vi "Start Download.vi"(5 "Overall Status":refnum<vi>, 7 "Itemized Status":refnum<vi>, 8 "Error In":errorcluster, 11 "Dependecy Config":T2) -> (0 "Error Out":errorcluster, 2 "Install State":T1(ring), 3 "Dependecy Config":T2)   [LabVIEW 2011, in "LVH-Toolbox.lvlib" / "Installer Tools.lvlib"]
uses:
  Installer Tools.lvlib
  Type Defs/Dependency Config.ctl
  Type Defs/Dependecy.ctl
  Common/Private/Web/Type Defs/Download Task.ctl
  Common/LVH-Common.lvlib
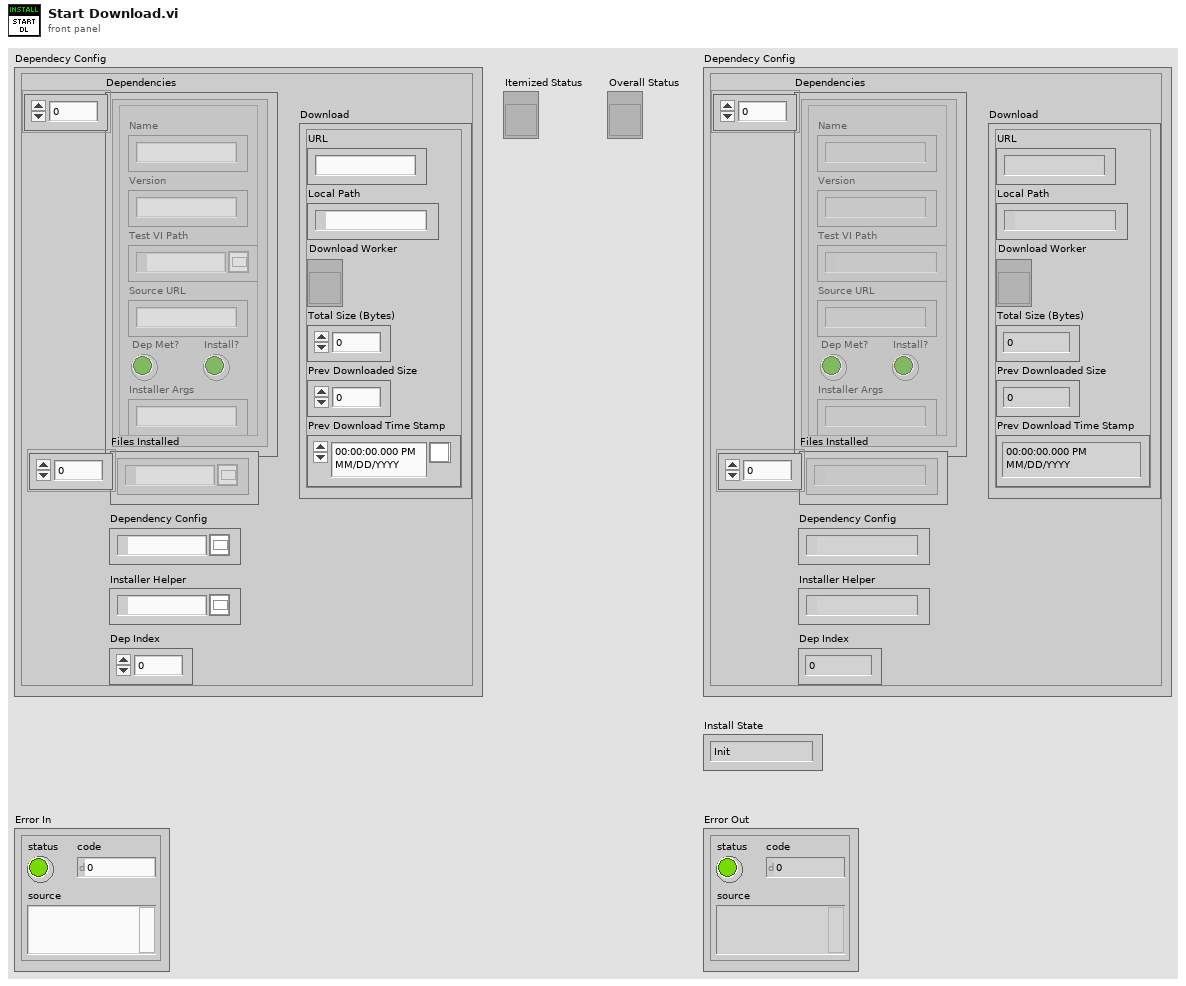
[diagram p1: front panel]
types:
  T1 = enum16{"Init", "Start DL", "Downloading", "DL Complete", "Done"}
  T2 = typedef "LVH-Toolbox.lvlib/Installer Tools.lvlib/Dependency Config.ctl" = cluster{"Dependencies":T3[], "Files Installed":path[], "Dependency Config":path, "Installer Helper":path, "Dep Index":i32, "Download":T4}
  T3 = typedef "LVH-Toolbox.lvlib/Installer Tools.lvlib/Dependecy.ctl" = cluster{"Name":string, "Version":string, "Test VI Path":path, "Source URL":string, "Dep Met?":bool, "Install?":bool, "Installer Args":string}
  T4 = typedef "LVH-Toolbox.lvlib/LVH-Common.lvlib/Download Task.ctl" = cluster{"URL":string, "Local Path":path, "Download Worker":refnum<vi>, "Total Size (Bytes)":u64, "Prev Downloaded Size":u64, "Prev Download Time Stamp":timestamp}
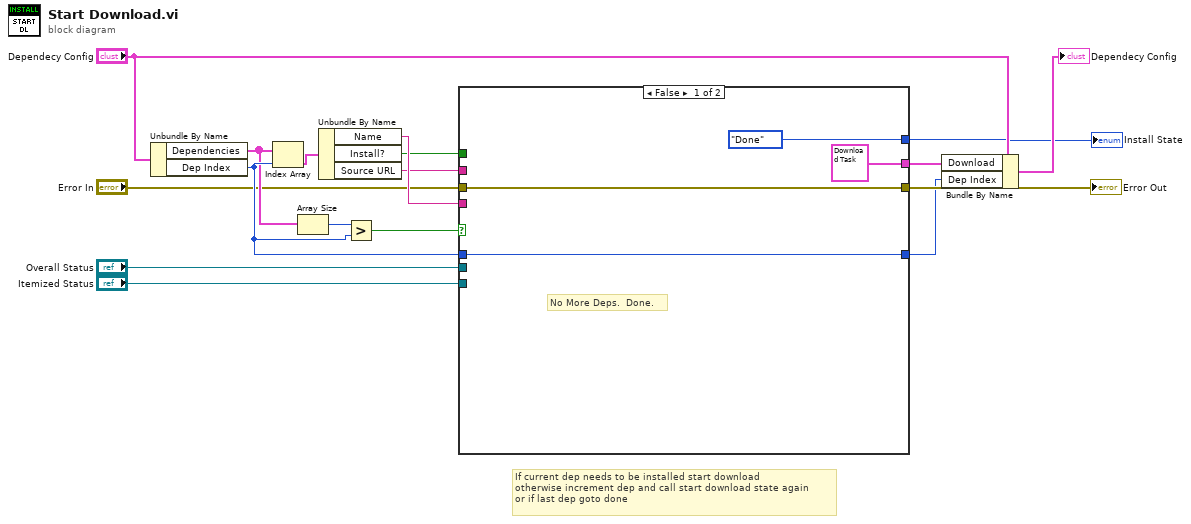
[diagram p0: block diagram]
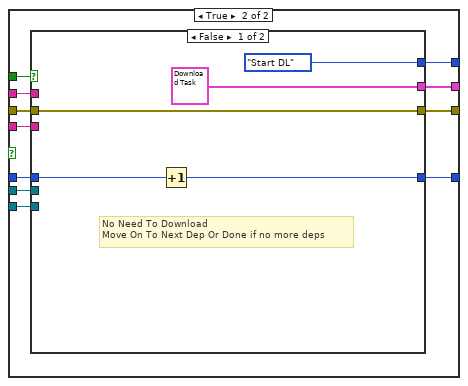
[diagram p2: hidden frame]
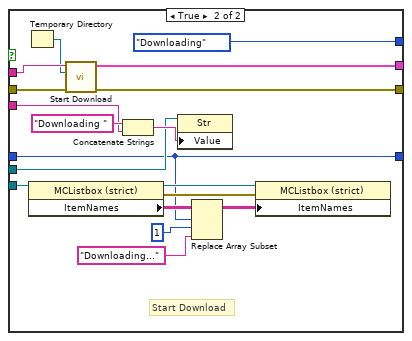
[diagram p3: hidden frame]
diagram:
  # "If current dep needs to be installed start download\notherwise increment dep and call start download state again \nor if last dep goto done"
  n1 = Unbundle By Name("Dependecy Config") -> ("Dependencies"=w13:T3[], "Dep Index"=w17:i32)
  n2 = Index Array(array=w13, index=w17) -> (element=w10:T3)
  n3 = Array Size(array=w13) -> (size(s)=w14:i32)
  n4 = Unbundle By Name(w10) -> ("Name"=w16:string, "Install?"=w11:bool, "Source URL"=w12:string)
  n5 = Greater?(x=w14, y=w17) -> (0:w15:bool)
  n6 = case shown="False" w15 {
    tunnel: "Error In" -> [w21 w32]
    tunnel: [w21 w31] -> w9
    tunnel: [T4 {"URL"="", "Local Path"=path "", "Download Worker"=refnum, "Total Size (Bytes)"=0, "Prev Downloaded Size"=0, "Prev Download Time Stamp"=timestamp(0 s since 1904-01-01)} ("Download") w30] -> w5
    tunnel: [T1."Done" ("Install State") w29] -> w2
    tunnel: w11 -> [_ w28]
    tunnel: w12 -> [_ w27]
    tunnel: w17 -> [w18 w26]
    tunnel: w16 -> [_ w25]
    tunnel: "Overall Status" -> [_ w24]
    tunnel: "Itemized Status" -> [_ w23]
    tunnel: [w18 w22] -> w1
    frame False {
      # "No More Deps.  Done."
    }
    frame True {
      n7 = case shown="False" w28 {
        tunnel: w27 -> [_ w55]
        tunnel: w32 -> [w37 w54]
        tunnel: [w37 w53] -> w31
        tunnel: [T4 {"URL"="", "Local Path"=path "", "Download Worker"=refnum, "Total Size (Bytes)"=0, "Prev Downloaded Size"=0, "Prev Download Time Stamp"=timestamp(0 s since 1904-01-01)} ("Download") w52] -> w30
        tunnel: w26 -> [w36 w38]
        tunnel: [T1."Start DL" ("Install State") T1."Downloading" ("Install State")] -> w29
        tunnel: w25 -> [_ w47]
        tunnel: w24 -> [_ w42]
        tunnel: w23 -> [_ w41]
        tunnel: [w33 w38] -> w22
        frame False {
          # "No Need To Download\nMove On To Next Dep Or Done if no more deps"
          n8 = Increment(x=w36) -> (x+1=w33:i32)
        }
        frame True {
          # "Start Download"
          n9 = Temporary Directory() -> (w50:path)
          n10 = property on="Property Node" class="MCListbox (strict)"(reference=w41) -> (reference out=w40:refnum<vi>, error out=w39:errorcluster, "ItemNames"=w46:string[][])  [unwired: 1 in]
          n11 = call "Start Download.vi"("Error In"=w54, "Download Directory"=w50, "URL"=w55) -> ("Error Out"=w53:errorcluster, "Download"=w52:T4)  [unwired: 7 in]
          n12 = Concatenate Strings("Downloading " ("string"), w47) -> (w48:string)
          n13 = property class="Str"(reference=w42, "Value"=w48) -> ()  [unwired: 1 in, 2 out]
          n14 = Replace Array Subset(array=w46, new element="Downloading..." ("new element/subarray"), index (row)=w38, index (col)=1 ("disabled index (row)")) -> (w45:string[][])
          n15 = property on="Property Node" class="MCListbox (strict)"(reference=w40, error in=w39, "ItemNames"=w45) -> ()  [unwired: 2 out]
        }
      }
    }
  }
  "Error Out" <- w9
  "Install State" <- w2
  n16 = Bundle By Name(cluster="Dependecy Config", "Download"=w5, "Dep Index"=w1) -> (→"Dependecy Config":T2)
